vi "Configure dBm.vi"(0 "VISA resource name":refnum<visa-resource-name>, 5 "error in (no error)":errorcluster, 6 "State":bool, 9 "dBm Reference":dbl=600.0) -> (14 "VISA resource name out":refnum<visa-resource-name>, 19 "error out":errorcluster)   [LabVIEW 2020, in "Keithley 2100 Series.lvlib"]
doc: "Definition:\nWith dBm selected, a voltage measurement is displayed as the level of power, relative to 1 milliwatt, dissipated through a reference resistance. The reference resistance is adjustable in KE2100. The calculation of dBm is defined as below:\n\n dBm = 10log(V^2in/Zref)/1mW\n\nNote: in V is the input signal voltage. ref Z is the reference resistance.\nNote: Change of reference resistance will not affect the stored relative reference value.\n\n.. The Zref is adjustable with a range from 50O to 8000 O. The default\nvalue is 600 O.\n.. The user selected reference value is stored in a volatile memory and will be cleared after the multimeter has been power-off.\n.. This feature is available for DCV and ACV only.\n\nHow to set the reference resistance:\nUser can set the reference resistance either through the front panel operation or the remote interface operation.\n\nRemote Interface Operation:\n\nUse the following commands to enable dBm feature or to set the reference resistance:\n\nCALCulate:FUNCtion DBM\nCALCulate:STATe {OFF|ON}\nCALCulate:STATe?\nCALCulate:DBM:REFerence {<value>|MINimum|MAXimum}"
uses:
  Keithley 2100 Series.lvlib
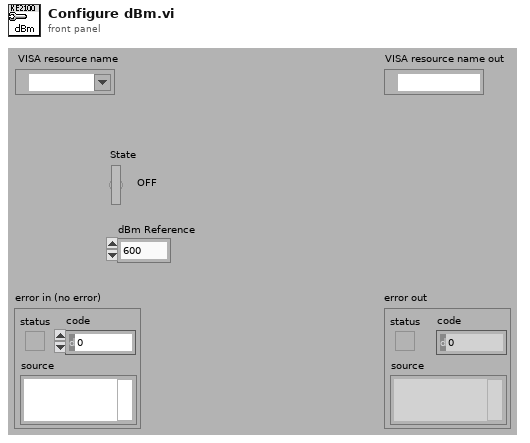
[diagram p1: front panel]
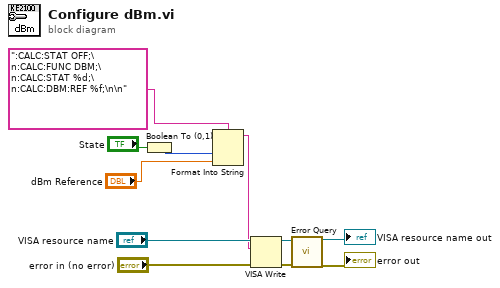
[diagram p0: block diagram]
diagram:
  n1 = Boolean To (0,1)(Boolean="State") -> (0, 1=w4:i16)
  n2 = Format Into String(format string=":CALC:STAT OFF;\n:CALC:FUNC DBM;\n:CALC:STAT %d;\n:CALC:DBM:REF %f;\n\n", w4, "dBm Reference") -> (resulting string=w5:string)  [unwired: 2 in, 1 out]
  n3 = VISA Write(VISA resource name="VISA resource name", write buffer=w5, error in (no error)="error in (no error)") -> (VISA resource name out=w10:refnum<visa-resource-name>, error out=w11:errorcluster)  [unwired: 1 out]
  n4 = call "Error Query.vi"("VISA resource name"=w10, "error in (no error)"=w11) -> ("VISA resource name out"=→"VISA resource name out":refnum<visa-resource-name>, "error out"=→"error out":errorcluster)  [unwired: 14 in, 2 out]
